vi "plot_obstacles.vi"(9 "MapDistanceInfo":T1 {"Top Left Pixel UTM"."North" format="%#_10f"; "Top Left Pixel UTM"."East" format="%#_8f"; "Bottom Right Pixel UTM"."North" format="%#_10f"; "Bottom Right Pixel UTM"."East" format="%#_8f"}, 10 "Current Obstacles":refnum<class "Obstacle.lvclass">[](array[class]), 11 "Map in":T3) -> (1 "MapDistanceInfo OUT":T1 {"Top Left Pixel UTM"."North" format="%#_10f"; "Top Left Pixel UTM"."East" format="%#_8f"; "Bottom Right Pixel UTM"."North" format="%#_10f"; "Bottom Right Pixel UTM"."East" format="%#_8f"}, 3 "Map Out":T3)   [LabVIEW 2013]
uses:
  <vilib>/vision/Image Controls.llb/IMAQ Image.ctl
  TypeDef/map_metadata.ctl
  cRIO_Code/Data/TypeDefs/UTM Location.ctl
  cRIO_Code/Logic/Classes/Obstacle/Obstacle.lvclass
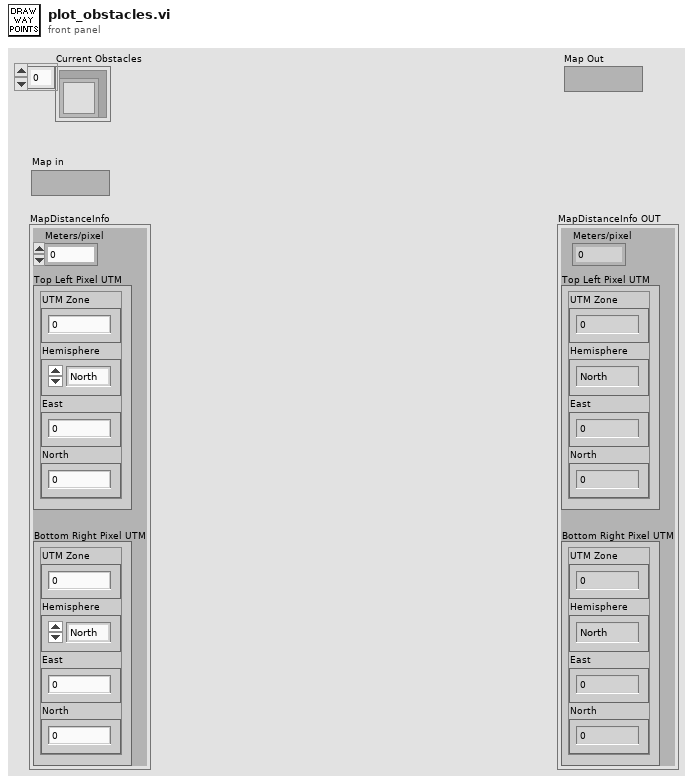
[diagram p1: front panel]
types:
  T1 = typedef "map_metadata.ctl" = cluster{"Meters/pixel":dbl, "Top Left Pixel UTM":T2, "Bottom Right Pixel UTM":T2}
  T2 = typedef "UTM Location.ctl" = cluster{"UTM Zone":dbl, "Hemisphere":enum16{"North", "South"}, "East":dbl, "North":dbl}
  T3 = typedef "IMAQ Image.ctl" = refnum<image>
  T4 = cluster{"UTM Obstacle Point 2":T2, "UTM Obstacle Point 1":T2}[]
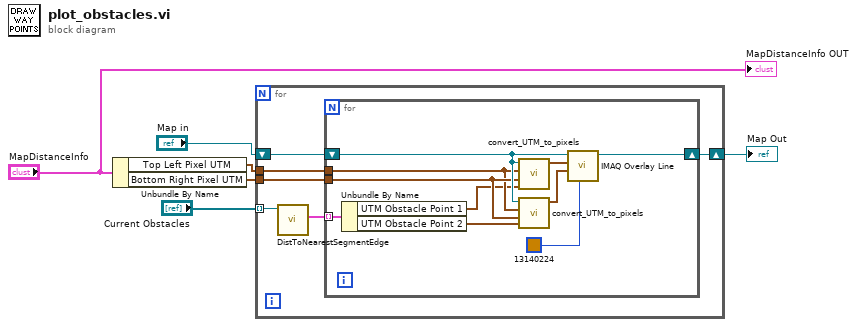
[diagram p0: block diagram]
diagram:
  n1 = Unbundle By Name("MapDistanceInfo") -> ("Top Left Pixel UTM"=w3:T2, "Bottom Right Pixel UTM"=w2:T2)
  n2 = for {
    tunnel: "Current Obstacles" -> [w12] mode=indexing
    shift-right: [w10] -> w1
    shift-left: "Map in" -> [w9]
    tunnel: w3 -> [w8]
    tunnel: w2 -> [w7]
    n3 = call "DistToNearestSegmentEdge.vi"("Obstacle.lvclass"=w12) -> ("List of Line Segments in Obstacle"=w11:T4)  [unwired: 9 in, 1 out]
    n4 = for {
      tunnel: w11 -> [w18] mode=indexing
      shift-right: [w22] -> w10
      shift-left: w9 -> [w21]
      tunnel: w8 -> [w19]
      tunnel: w7 -> [w20]
      n5 = Unbundle By Name(w18) -> ("UTM Obstacle Point 1"=w17:T2, "UTM Obstacle Point 2"=w16:T2)
      n6 = call "convert_UTM_to_pixels.vi"("UTM position of Boat"=w17, "Bottom Right Pixel UTM"=w20, "Top Left Pixel UTM"=w19, "Map in"=w21) -> ("Position"=w15:cluster{"X":i32, "Y":i32})  [unwired: 6 in, 1 out]
      n7 = call "convert_UTM_to_pixels.vi"("UTM position of Boat"=w16, "Bottom Right Pixel UTM"=w20, "Top Left Pixel UTM"=w19, "Map in"=w21) -> ("Position"=w14:cluster{"X":i32, "Y":i32})  [unwired: 6 in, 1 out]
      n8 = call "IMAQ Overlay Line"("Color"=u32 13140224, "End Point"=w14, "Start Point"=w15, "Image"=w21) -> ("Image Out"=w22:T3)  [unwired: 6 in, 1 out]
    }
  }
  "Map Out" <- w1
  "MapDistanceInfo OUT" <- "MapDistanceInfo"
